vi "Encode Pretty.vi"(11 "Pretty Indent (-1=None)":i32=-1) -> (1 "EOL":string, 2 "key-value gap":string, 3 "prefix":string)   [LabVIEW 2019, in "JSON.lvlib"]
doc: "Calculates the pretty print whitespace if <b>Pretty Indent</b> is greater or equal to zero. Otherwise, this compacts the JSON string.\n\nCreated by: Ryan Pacini"
uses:
  JSON.lvlib
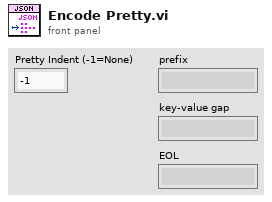
[diagram p1: front panel]
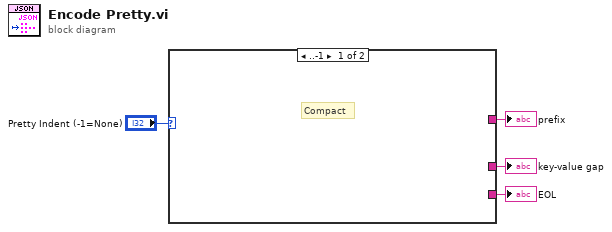
[diagram p0: block diagram]
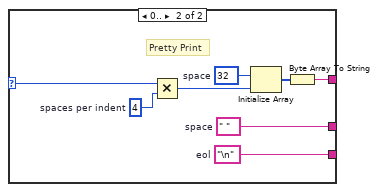
[diagram p2: hidden frame]
diagram:
  n1 = case shown="..-1" "Pretty Indent (-1=None)" {
    selector: "Pretty Indent (-1=None)" -> [_ w9]
    tunnel: [_ w8] -> w3
    tunnel: [_ w6] -> w2
    tunnel: [_ w5] -> w1
    frame ..-1 {
      # "Compact"
    }
    frame 0.. {
      w5 = "\n"  # eol
      w6 = " "  # space
      w10 = 4  # spaces per indent
      w7 = u8 32  # space
      # "Pretty Print"
      n2 = Multiply(x=w9, y=w10) -> (x*y=w11:i32)
      n3 = Initialize Array(w7, w11) -> (w12:u8[])
      n4 = Byte Array To String(unsigned byte array=w12) -> (string=w8:string)
    }
  }
  "prefix" <- w3
  "key-value gap" <- w2
  "EOL" <- w1
